vi "SplineParam_StackGet.vi"(11 "InputStack":T1) -> (1 "T1":dbl, 3 "T0":dbl)   [LabVIEW 2019, in "Trajectory_Library.lvlib"]
doc: "Internal routine used by SplineParam_Spline_T0_T1. This routine gets, but does not remove, the item from the top of the stack.\n\nParameters:\n - InputStack - Stack data structure\n\nReturns:\n - T0\n - T1"
uses:
  Trajectory_Library.lvlib
  TypeDef/PARAM_STACK.ctl
  TypeDef/PARAM_STACK_ITEM.ctl
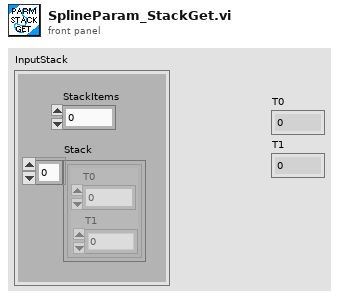
[diagram p1: front panel]
types:
  T1 = typedef "Trajectory_Library.lvlib/PARAM_STACK.ctl" = cluster{"StackItems":i32, "Stack":T2[]}
  T2 = typedef "Trajectory_Library.lvlib/PARAM_STACK_ITEM.ctl" = cluster{"T0":dbl, "T1":dbl}
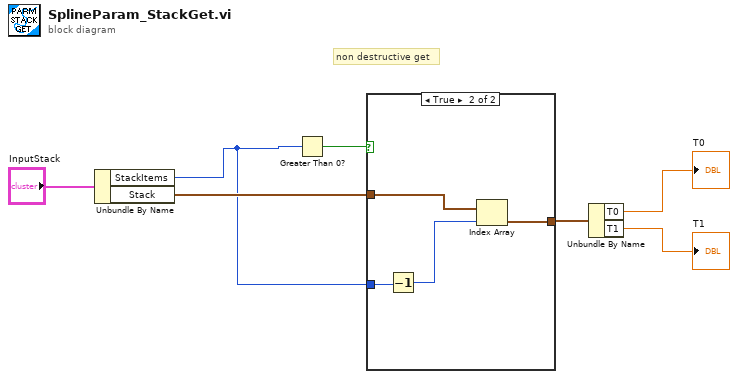
[diagram p0: block diagram]
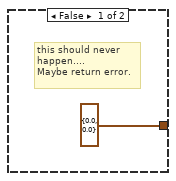
[diagram p2: hidden frame]
diagram:
  # "non destructive get"
  n1 = Unbundle By Name("InputStack") -> ("StackItems"=w4:i32, "Stack"=w5:T2[])
  n2 = Greater Than 0?(x=w4) -> (x > 0?=w6:bool)
  n3 = case shown="True" w6 {
    tunnel: w5 -> [_ w10]
    tunnel: w4 -> [_ w12]
    tunnel: [T2 {"T0"=0.0, "T1"=0.0} ("PARAM_STACK") w9] -> w3
    frame False {
      # "this should never \nhappen....\nMaybe return error."
    }
    frame True {
      n4 = Decrement(x=w12) -> (x-1=w11:i32)
      n5 = Index Array(array=w10, index=w11) -> (element=w9:T2)
    }
  }
  n6 = Unbundle By Name(w3) -> ("T0"=→"T0":dbl, "T1"=→"T1":dbl)
